vi "Write LibraryDirectories.vi"(10 "LibraryDirectories":T1, 11 "Project in":refnum<class "Project.lvclass">) -> (3 "Project out":refnum<class "Project.lvclass">)   [LabVIEW 2016, in "Project.lvclass"]
uses:
  Project.lvclass
  Typedefs/LibraryDirectories.ctl
  Project.lvclass/Project.ctl
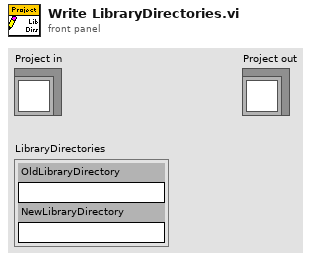
[diagram p1: front panel]
types:
  T1 = typedef "LibraryDirectories.ctl" = cluster{"OldLibraryDirectory":string, "NewLibraryDirectory":string}
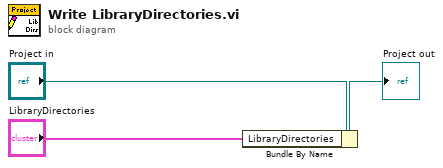
[diagram p0: block diagram]
diagram:
  n1 = Bundle By Name(cluster="Project in", "LibraryDirectories"="LibraryDirectories") -> (→"Project out":refnum<class "Project.lvclass">)
